vi "Get Node ID.vi"(11 "Node Path":path) -> (3 "Node ID":string)   [LabVIEW 2020, in "SimpleDependencyInspector.lvlib"]
uses:
  SimpleDependencyInspector.lvlib
  FGV Functions--enum.ctl
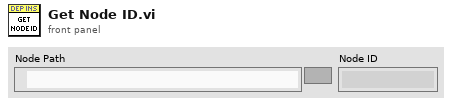
[diagram p1: front panel]
types:
  T1 = typedef "SimpleDependencyInspector.lvlib/FGV Functions--enum.ctl" = enum16{"Initialize", "Get Node ID", "Set Node ID"}
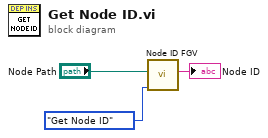
[diagram p0: block diagram]
diagram:
  n1 = call "Node ID FGV.vi"("Initialize"=FGV_Functions--enum."Get Node ID", "Node Path"="Node Path") -> ("Node ID"=→"Node ID":string)  [unwired: 7 in, 2 out]
